vi "Delete accidental time series.vi"(8 "error in (no error)":errorcluster, 11 "Logging queue element in":T1={"Imaging Protocol"=enum."Live Imaging", "Number of Trials"=0, "Frame Size"=512, "# Averaged frames"=0, "Dwell time (us)"=0.0, "Index of Z-plane"=0, "Timelapse?"=FALSE, "Logging process is active"=FALSE, "Speed logging enabled"=FALSE, "tdms file ref"=refnum, "path"=path "", "Trial Number"=0, "Expected # points acquired"=FALSE, "Manually stopped"=FALSE, "Ch0 data"=[], "Ch1 data"=[], "Ref Data"=[], "Last trial"=FALSE, "Ref Dwell time (us)"=0.0, "# Ref Averaged frames"=0, "Ref X Length"=0, "Ref Y Length"=0, "Points acquired"={"Ch0 last trial"=0, "Ch1 last trial"=0, "All trials"=0}} {"Ref Dwell time (us)" format="%#.6g"; "Frame Size" items=["100X100"=100, "128X128"=128, "200X200"=200, "256X256"=256, "512X512"=512, "1024x1024"=1024, "2048x2048"=2048]; "Dwell time (us)" format="%#.6g"}) -> ()   [LabVIEW 2017]
uses:
  Typedefs/Logging queue element.ctl
  Typedefs/Imaging Protocols enum.ctl
  Typedefs/Frame Size.ctl
  Typedefs/Acquired points count.ctl
  Global Variables/General Globals.vi
panel:
  out "Last experiment folder path":path
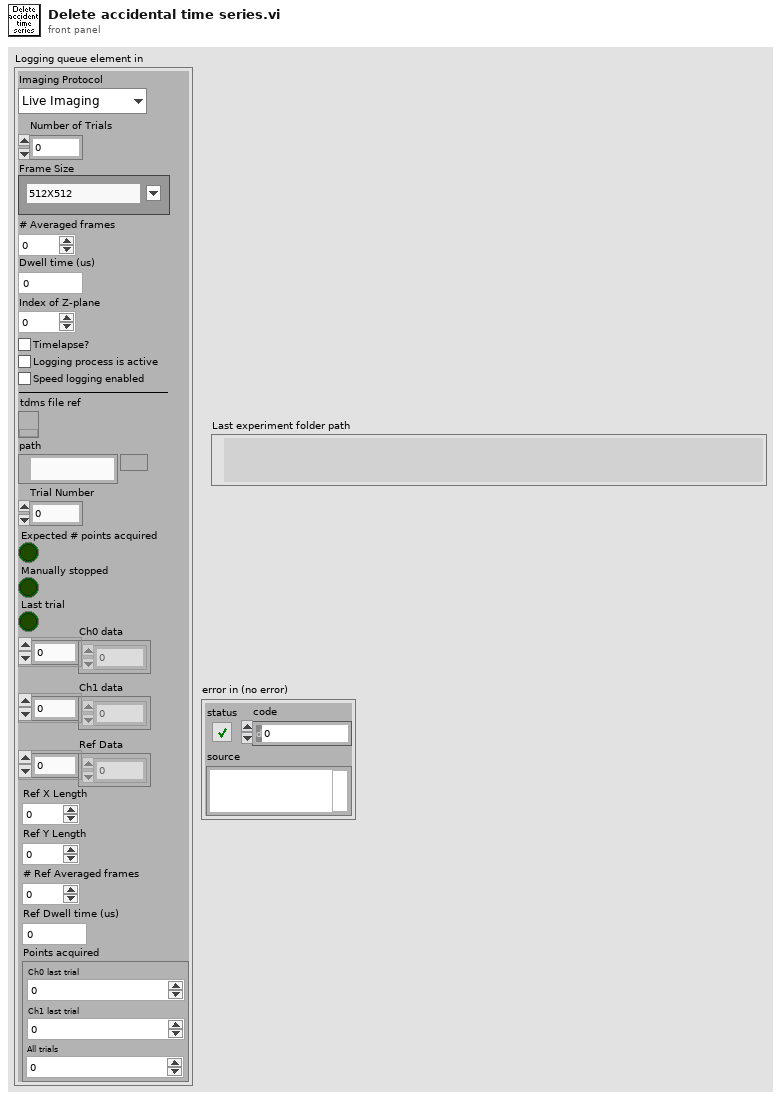
[diagram p1: front panel]
types:
  T1 = typedef "Logging queue element.ctl" = cluster{"Imaging Protocol":T2, "Number of Trials":u16, "Frame Size":T3, "# Averaged frames":u16, "Dwell time (us)":dbl, "Index of Z-plane":i32, "Timelapse?":bool, "Logging process is active":bool, "Speed logging enabled":bool, "tdms file ref":refnum<k34>, "path":path, "Trial Number":i32, "Expected # points acquired":bool, "Manually stopped":bool, "Ch0 data":u32[], "Ch1 data":u32[], "Ref Data":u32[], "Last trial":bool, "Ref Dwell time (us)":dbl, "# Ref Averaged frames":u16, "Ref X Length":u16, "Ref Y Length":u16, "Points acquired":T4}
  T2 = typedef "Imaging Protocols enum.ctl" = enum16{"AOL Z-Stack", "Motor Z Stack", "Functional Acquisition", "Single Plane Acquisition", "Volume Acquisition", "Live Imaging", "Live Plane Imaging", "Live Volume Imaging"}
  T3 = typedef "Frame Size.ctl" = u16
  T4 = typedef "Acquired points count.ctl" = cluster{"Ch0 last trial":u64, "Ch1 last trial":u64, "All trials":u64}
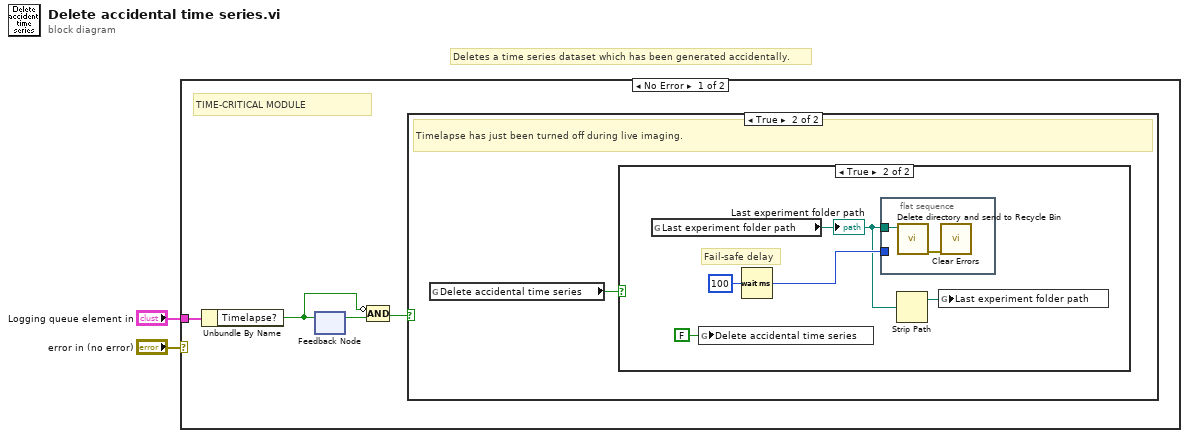
[diagram p0: block diagram]
diagram:
  # "Deletes a time series dataset which has been generated accidentally."
  n1 = case shown="No Error" "error in (no error)" {
    tunnel: "Logging queue element in" -> [w6 _]
    frame No Error {
      # "TIME-CRITICAL MODULE"
      n2 = Unbundle By Name(w6) -> ("Timelapse?"=w5:bool)
      n3 = feedback #1() -> (w4:bool)  [unwired: 1 in]
      n4 = feedback-in #1(w5) -> ()
      n5 = Compound Arithmetic op=AND(invert w5, w4) -> (w3:bool)
      n6 = case shown="True" w3 {
        frame False {
          # "Not stopped"
        }
        frame True {
          # "Timelapse has just been turned off during live imaging."
          n7 = global read "General Globals.vi" "Delete accidental time series"() -> (w7:bool)
          n8 = case shown="True" w7 {
            frame False {
            }
            frame True {
              # "Fail-safe delay"
              n9 = global read "General Globals.vi" "Last experiment folder path"() -> (w9:path)
              "Last experiment folder path" <- w9
              n10 = global write "General Globals.vi" "Delete accidental time series"(FALSE ("Delete accidental time series")) -> ()
              n11 = Wait (ms)(milliseconds to wait=u32 100) -> (millisecond timer value=w10:u32)
              n12 = flat-sequence {
                tunnel: w9 -> [w14]
                tunnel: w10 -> [_]
                frame #0 {
                  n13 = call <userlib>:"Delete directory and send to Recycle Bin.vi"("Directory to Recycle"=w14) -> ("error out"=w13:errorcluster)  [unwired: 10 in]
                  n14 = call <vilib>:"Clear Errors.vi"("error in (no error)"=w13) -> ()  [unwired: 5 in, 2 out]
                }
              }
              n15 = Strip Path(path=w9) -> (stripped path=w8:path)  [unwired: 1 out]
              n16 = global write "General Globals.vi" "Last experiment folder path"(w8) -> ()
            }
          }
        }
      }
    }
    frame Error {
    }
  }
